vi "commandHandler.vi"(8 "error in (no error)":errorcluster, 10 "Camera":refnum<class>, 11 "CameraNetworkClient in":refnum<class "CameraNetworkServer.lvclass">) -> (0 "error out":errorcluster, 3 "CameraNetworkClient out":refnum<class "CameraNetworkServer.lvclass">)   [LabVIEW 2009, in "Hardware.lvlib" / "HWControllers.lvlib" / "CameraNetworkServer.lvclass"]
uses:
  CameraNetworkServer.lvclass
  Channels/Camera/Camera/Camera.lvclass
  CameraNetworkServer.lvclass/CameraNetworkServer.ctl
  Tools/CameraSettings/CamaraSettings.lvclass
  NetworkClient/NetworkServer.lvclass
panel:
  out "fps":dbl
  out "elements":T1(array[cluster])
  out "element":T2
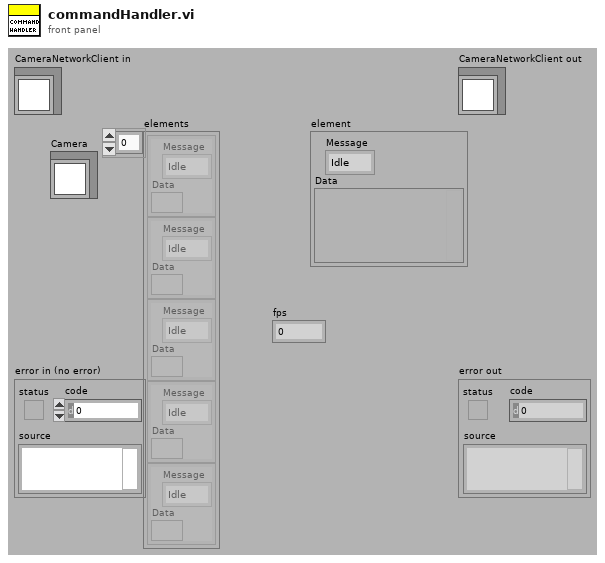
[diagram p1: front panel]
types:
  T1 = cluster{"Message":enum16{"Idle", "initialise", "configureAcquisition", "setTemperature", "getTemperature", "start", "stop", "sendImage", "close", "error", "ExitApp"}, "Data":variant}[]
  T2 = cluster{"Message":enum16{"Idle", "initialise", "configureAcquisition", "setTemperature", "getTemperature", "start", "stop", "sendImage", "close", "error", "ExitApp", "getAcquisitionStatus"}, "Data":variant}
  T3 = cluster{"CamaraSettings":refnum<class "CamaraSettings.lvclass">, "saveImages?":bool, "imagePaths":path[], "number of Images":i32}
  T4 = cluster{"Message":enum16{"Idle", "initialise", "configureAcquisition", "setTemperature", "getTemperature", "start", "stop", "sendImage", "close", "error", "ExitApp", "getAcquisitionStatus"}, bool}
  T5 = cluster{"cameraType":string, "imageName":string, "saved":string, "analysisType":string, "I16bit image data":i16[][], "path":path}
  T6 = cluster{"Message":enum16{"Idle", "initialise", "configureAcquisition", "setTemperature", "getTemperature", "start", "stop", "sendImage", "close", "error", "ExitApp", "getAcquisitionStatus"}, bool}[]
  T7 = cluster{"Message":enum16{"Idle", "initialise", "configureAcquisition", "setTemperature", "getTemperature", "start", "stop", "sendImage", "close", "error", "ExitApp"}, bool}
  T8 = enum16{"Idle", "initialise", "configureAcquisition", "setTemperature", "getTemperature", "start", "stop", "sendImage", "close", "error", "ExitApp"}
  T9 = cluster{"Message":enum16{"Idle", "initialise", "configureAcquisition", "setTemperature", "getTemperature", "start", "stop", "sendImage", "close", "error", "ExitApp", "getAcquisitionStatus"}, "Data":variant}[]
  T10 = enum16{"Idle", "initialise", "configureAcquisition", "setTemperature", "getTemperature", "start", "stop", "sendImage", "close", "error", "ExitApp", "getAcquisitionStatus"}
  T11 = cluster{"Message":enum16{"Idle", "initialise", "configureAcquisition", "setTemperature", "getTemperature", "start", "stop", "sendImage", "close", "error", "ExitApp"}, bool}[]
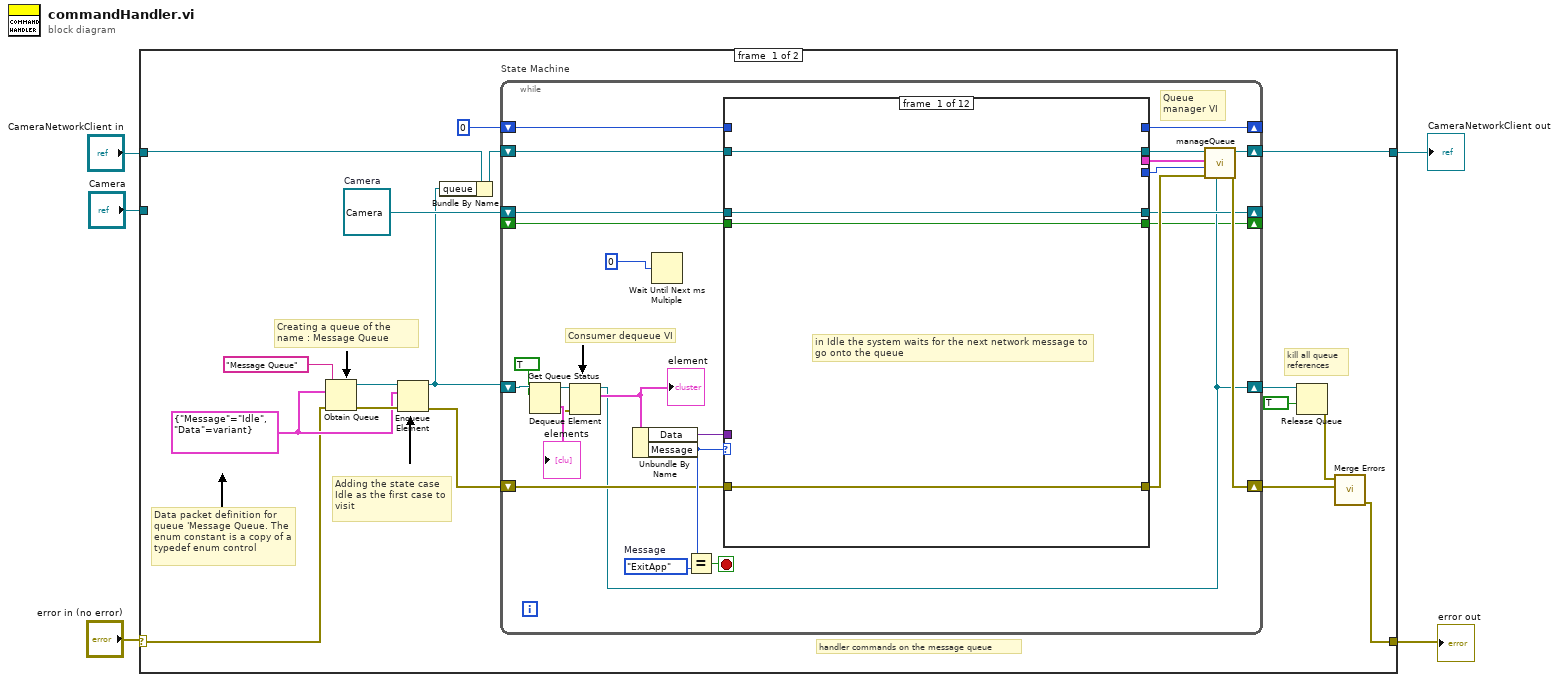
[diagram p0: block diagram]
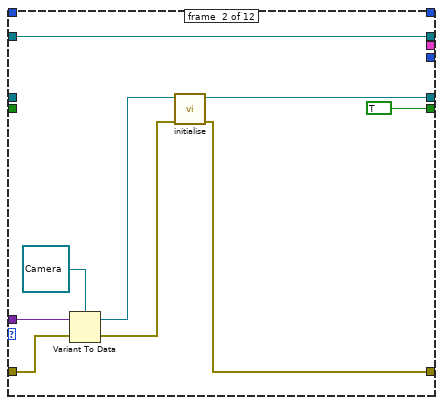
[diagram p2: hidden frame]
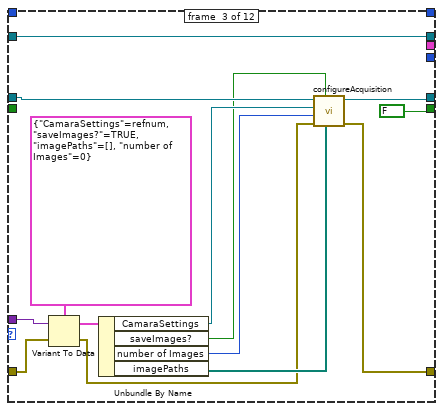
[diagram p3: hidden frame]
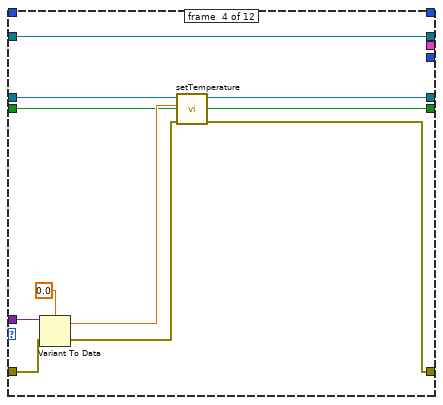
[diagram p4: hidden frame]
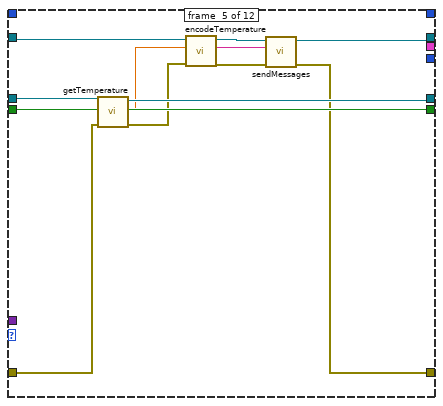
[diagram p5: hidden frame]
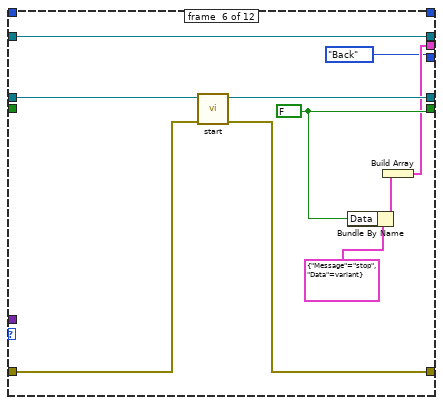
[diagram p6: hidden frame]
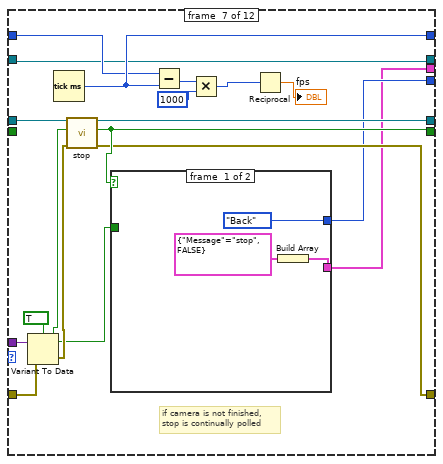
[diagram p7: hidden frame]
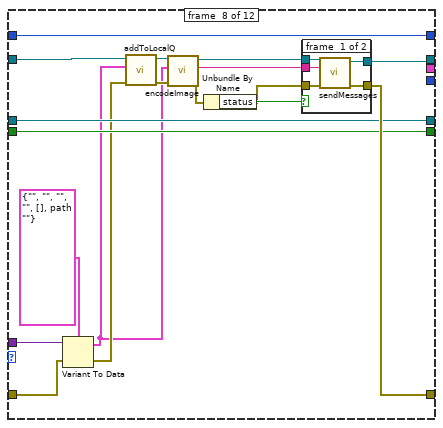
[diagram p9: hidden frame]
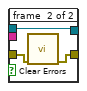
[diagram p10: hidden frame]
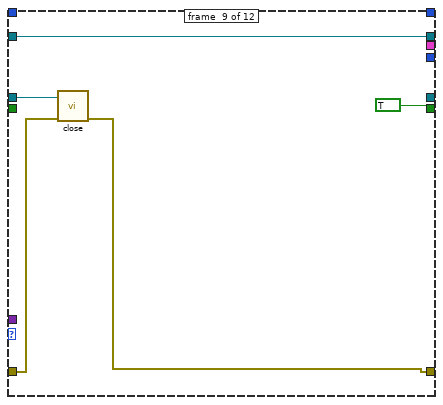
[diagram p11: hidden frame]
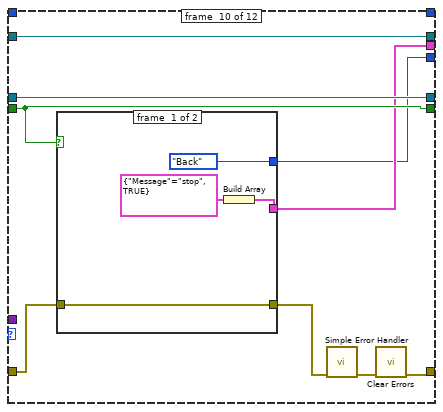
[diagram p12: hidden frame]
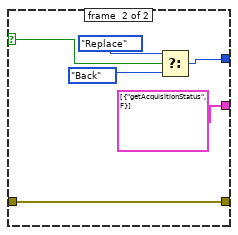
[diagram p13: hidden frame]
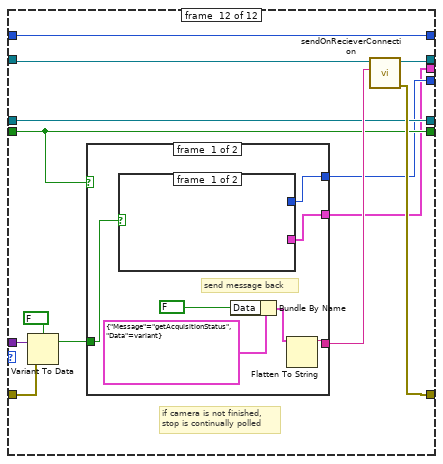
[diagram p15: hidden frame]
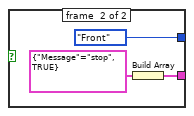
[diagram p16: hidden frame]
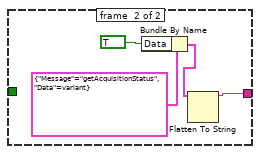
[diagram p17: hidden frame]
diagram:
  n1 = case shown="No Error" "error in (no error)" {
    selector: "error in (no error)" -> [w14 w210]
    tunnel: [w11 w210] -> w3
    tunnel: [w15 w209] -> w2
    tunnel: "CameraNetworkClient in" -> [w10 w209]
    tunnel: "Camera" -> [_ _]
    frame #0 {
      w8 = refnum<class "Camera.lvclass"> refnum  # Camera
      w17 = T2 {"Message"=enum."Idle", "Data"=variant}
      # "handler commands on the message queue"
      # "kill all queue \nreferences"
      # "Data packet definition for queue 'Message Queue. The enum constant is a copy of a typedef enum control"
      # "Adding the state case Idle as the first case to visit"
      # "Creating a queue of the name : Message Queue"
      n2 = Obtain Queue(name (unnamed)="Message Queue" ("Queue Name"), element data type=w17, error in (no error)=w14) -> (queue out=w20:refnum<queue>, error out=w21:errorcluster)  [unwired: 2 in, 1 out]
      n3 = Enqueue Element(queue=w20, element=w17, error in (no error)=w21) -> (queue out=w6:refnum<queue>, error out=w16:errorcluster)  [unwired: 1 in, 1 out]
      n4 = Bundle By Name(cluster=w10, "queue"=w6) -> (w9:refnum<class "CameraNetworkServer.lvclass">)
      n5 = while "State Machine" {
        shift-right: [w39] -> w12
        shift-left: w16 -> [w46]
        shift-right: [w34] -> w18
        shift-left: w6 -> [w30]
        shift-right: [w41] -> w15
        shift-left: w9 -> [w43]
        shift-right: [w36] -> _
        shift-left: w8 -> [w35]
        shift-right: [w33] -> _
        shift-left: _ -> [w32]
        shift-right: [w26] -> _
        shift-left: 0 -> [w25]
        stop <- w45 stop-if-true
        w37 = T8."ExitApp"  # Message
        # "Queue manager VI"
        # "Consumer dequeue VI"
        n6 = Get Queue Status(queue=w30, return elements? (F)=TRUE) -> (queue out=w31:refnum<queue>, error out=w27:errorcluster, elements=→"elements":T9)  [unwired: 1 in, 5 out]
        n7 = Dequeue Element(queue=w31, error in (no error)=w27) -> (queue out=w34:refnum<queue>, element=w44:T2)  [unwired: 1 in, 2 out]
        "element" <- w44
        n8 = Unbundle By Name(w44) -> ("Data"=w48:variant, "Message"=w47:T10)
        n9 = Wait Until Next ms Multiple(millisecond multiple=0) -> ()  [unwired: 1 out]
        n10 = Equal?(x=w47, y=w37) -> (x = y?=w45:bool)
        n11 = case shown="\"sendImage\"" w47 {
          tunnel: w46 -> [w50 w56 w73 w81 w95 w104 w120 w139 w156 w160 w178 w192]
          tunnel: [w50 w59 w63 w77 w86 w103 w110 w144 w157 w164 w178 w187] -> w40
          tunnel: w48 -> [_ w57 w74 w82 _ _ w122 w140 _ _ _ w194]
          tunnel: w43 -> [w52 w61 w75 w85 w93 w107 w111 w136 w154 w167 w181 w190]
          tunnel: [w52 w61 w75 w85 w91 w107 w111 w145 w154 w167 w181 w189] -> w42
          tunnel: [_ _ _ _ _ enum16{"Back", "Front", "Replace"}."Back" ("FNs") w109 _ _ w161 _ w183] -> w38
          tunnel: [_ _ _ _ _ w99 w108 _ _ w162 _ w182] -> w24
          tunnel: [w51 w60 w69 w83 w96 w105 w124 w141 _ w166 w179 w185] -> w36
          tunnel: w35 -> [w51 _ w70 w84 w97 w106 w125 w141 w158 w166 w179 w185]
          tunnel: [w49 TRUE ("stopped?") FALSE w76 w94 w101 w123 w138 TRUE w163 w180 w184] -> w33
          tunnel: w32 -> [w49 _ _ w76 w94 _ _ w138 _ w163 w180 w184]
          tunnel: [_ _ _ _ _ _ w117 w137 _ _ _ w186] -> w26
          tunnel: w25 -> [_ _ _ _ _ _ w116 w137 _ _ _ w186]
          frame #0 {
            # "in Idle the system waits for the next network message to \ngo onto the queue"
          }
          frame #1 {
            n12 = Variant To Data(error in=w56, Variant=w57, type=refnum<class "Camera.lvclass"> refnum ("Hardware:Channels.lvlib:Camera.lvclass")) -> (error out=w55:errorcluster, data=w53:refnum<class "Camera.lvclass">)
            n13 = call-dynamic "initialise.vi"("error in (no error)"=w55, "Camera in"=w53) -> ("error out"=w59:errorcluster, "Camera out"=w60:refnum<class "Camera.lvclass">)  [unwired: 8 in]
          }
          frame #2 {
            n14 = Variant To Data(error in=w73, Variant=w74, type=T3 {"CamaraSettings"=refnum, "saveImages?"=TRUE, "imagePaths"=[], "number of Images"=0}) -> (error out=w64:errorcluster, data=w71:T3)
            n15 = Unbundle By Name(w71) -> ("CamaraSettings"=w68:refnum<class "CamaraSettings.lvclass">, "saveImages?"=w67:bool, "number of Images"=w66:i32, "imagePaths"=w65:path[])
            n16 = call-dynamic "configureAcquisition.vi"("imagePaths"=w65, "saveImages?"=w67, "error in (no error)"=w64, "number of Images"=w66, "CameraSettings"=w68, "Camera in"=w70) -> ("error out"=w63:errorcluster, "Camera out"=w69:refnum<class "Camera.lvclass">)  [unwired: 4 in]
          }
          frame #3 {
            n17 = Variant To Data(error in=w81, Variant=w82, type=0.0 ("setPoint")) -> (error out=w80:errorcluster, data=w78:dbl)
            n18 = call-dynamic "setTemperature.vi"("error in (no error)"=w80, "setPoint"=w78, "Camera in"=w84) -> ("error out"=w77:errorcluster, "Camera out"=w83:refnum<class "Camera.lvclass">)  [unwired: 7 in]
          }
          frame #4 {
            n19 = call-dynamic "getTemperature.vi"("error in (no error)"=w95, "Camera in"=w97) -> ("error out"=w89:errorcluster, "temperature"=w88:dbl, "Camera out"=w96:refnum<class "Camera.lvclass">)  [unwired: 7 in]
            n20 = call "encodeTemperature.vi"("error in (no error)"=w89, "temperature"=w88, "CameraNetworkServer in"=w93) -> ("error out"=w90:errorcluster, "message"=w87:string, "CameraNetworkServer out"=w92:refnum<class "CameraNetworkServer.lvclass">)  [unwired: 6 in]
            n21 = call "sendMessages.vi"("error in (no error)"=w90, "messageString"=w87, "NetworkClient in"=w92) -> ("error out"=w86:errorcluster, "NetworkClient out"=w91:refnum<class "CameraNetworkServer.lvclass">)  [unwired: 7 in]
          }
          frame #5 {
            w101 = FALSE
            n22 = call-dynamic "start.vi"("error in (no error)"=w104, "Camera in"=w106) -> ("error out"=w103:errorcluster, "Camera out"=w105:refnum<class "Camera.lvclass">)  [unwired: 8 in]
            n23 = Bundle By Name(cluster=T2 {"Message"=enum."stop", "Data"=variant} ("element"), "Data"=w101) -> (w100:T2)
            n24 = Build Array(w100) -> (w99:T9)
          }
          frame #6 {
            # "if camera is not finished,\nstop is continually polled"
            n25 = Variant To Data(error in=w120, Variant=w122, type=TRUE) -> (error out=w119:errorcluster, data=w118:bool)
            n26 = Tick Count (ms)() -> (millisecond timer value=w117:u32)
            n27 = call-dynamic "stop.vi"("error in (no error)"=w119, "stop"=w118, "Camera in"=w125) -> ("error out"=w110:errorcluster, "stopped?"=w123:bool, "Camera out"=w124:refnum<class "Camera.lvclass">)  [unwired: 5 in, 1 out]
            n28 = case shown="False" w123 {
              tunnel: [w127 _] -> w108
              tunnel: [enum16{"Back", "Front", "Replace"}."Back" ("FNs") _] -> w109
              tunnel: w118 -> [_ _]
              frame #0 {
                n29 = Build Array(T4 {"Message"=enum."stop", FALSE}) -> (w127:T6)
              }
              frame #1 {
              }
            }
            n30 = Subtract(x=w116, y=w117) -> (x-y=w115:u32)
            n31 = Multiply(x=w115, y=1000) -> (x*y=w113:u32)
            n32 = Reciprocal(x=w113) -> (1/x=→"fps":dbl)
          }
          frame #7 {
            n33 = Variant To Data(error in=w139, Variant=w140, type=T5 {"cameraType"="", "imageName"="", "saved"="", "analysisType"="", "I16bit image data"=[], "path"=path ""} ("ImageData")) -> (error out=w133:errorcluster, data=w130:T5)
            n34 = call "addToLocalQ.vi"("error in (no error)"=w133, "ImageData"=w130, "CameraNetworkServer in"=w136) -> ("error out"=w134:errorcluster, "CameraNetworkServer out"=w135:refnum<class "CameraNetworkServer.lvclass">)  [unwired: 7 in]
            n35 = call "encodeImage.vi"("error in (no error)"=w134, "ImageData"=w130, "CameraNetworkClient in"=w135) -> ("error out"=w131:errorcluster, "MessageString"=w142:string, "CameraNetworkClient out"=w143:refnum<class "CameraNetworkServer.lvclass">)  [unwired: 6 in]
            n36 = Unbundle By Name(w131) -> ("status"=w132:bool)
            n37 = case shown="False" w132 {
              tunnel: [w150 w153] -> w145
              tunnel: [w149 w151] -> w144
              tunnel: w143 -> [w148 w153]
              tunnel: w142 -> [w147 _]
              tunnel: w131 -> [w146 w152]
              frame #0 {
                n38 = call "sendMessages.vi"("error in (no error)"=w146, "messageString"=w147, "NetworkClient in"=w148) -> ("error out"=w149:errorcluster, "NetworkClient out"=w150:refnum<class "CameraNetworkServer.lvclass">)  [unwired: 7 in]
              }
              frame #1 {
                n39 = call <vilib>:"Clear Errors.vi"("error in (no error)"=w152) -> ("error out"=w151:errorcluster)  [unwired: 6 in]
              }
            }
          }
          frame #8 {
            n40 = call-dynamic "close.vi"("error in (no error)"=w156, "Camera in"=w158) -> ("error out"=w157:errorcluster)  [unwired: 9 in]
          }
          frame #9 {
            n41 = case shown="True" w163 {
              selector: w163 -> [_ w172]
              tunnel: [w170 T6 [{"Message"=enum."getAcquisitionStatus", FALSE}]] -> w162
              tunnel: [enum16{"Back", "Front", "Replace"}."Back" ("FNs") w177] -> w161
              tunnel: w160 -> [w168 w173]
              tunnel: [w168 w173] -> w159
              frame #0 {
                n42 = Build Array(T4 {"Message"=enum."stop", TRUE}) -> (w170:T6)
              }
              frame #1 {
                n43 = Select(t=enum16{"Back", "Front", "Replace"}."Replace" ("FNs"), s=w172, f=enum16{"Back", "Front", "Replace"}."Back" ("FNs")) -> (s? t:f=w177:enum16{"Back", "Front", "Replace"})
              }
            }
            n44 = call <vilib>:"Simple Error Handler.vi"("error in (no error)"=w159) -> ("error out"=w165:errorcluster)  [unwired: 4 in, 4 out]
            n45 = call <vilib>:"Clear Errors.vi"("error in (no error)"=w165) -> ("error out"=w164:errorcluster)  [unwired: 6 in]
          }
          frame #10 {
          }
          frame #11 {
            # "if camera is not finished,\nstop is continually polled"
            n46 = Variant To Data(error in=w192, Variant=w194, type=FALSE) -> (data=w191:bool)  [unwired: 1 out]
            n47 = case shown="False" w184 {
              tunnel: [w201 _] -> w182
              tunnel: [w200 _] -> w183
              tunnel: w191 -> [w197 _]
              tunnel: [w199 w208] -> w188
              frame #0 {
                # "send message back"
                n48 = case shown="True" w197 {
                  tunnel: [_ w203] -> w201
                  tunnel: [_ enum16{"Back", "Front", "Replace"}."Front" ("FNs")] -> w200
                  frame #0 {
                  }
                  frame #1 {
                    n49 = Build Array(T7 {"Message"=enum."stop", TRUE}) -> (w203:T11)
                  }
                }
                n50 = Bundle By Name(cluster=T2 {"Message"=enum."getAcquisitionStatus", "Data"=variant}, "Data"=FALSE) -> (w195:T2)
                n51 = Flatten To String(anything=w195) -> (data string=w199:string)  [unwired: 3 in, 2 out]
              }
              frame #1 {
                n52 = Bundle By Name(cluster=T2 {"Message"=enum."getAcquisitionStatus", "Data"=variant}, "Data"=TRUE) -> (w205:T2)
                n53 = Flatten To String(anything=w205) -> (data string=w208:string)  [unwired: 3 in, 2 out]
              }
            }
            n54 = call "sendOnRecieverConnection.vi"("message"=w188, "NetworkServer in"=w190) -> ("error out"=w187:errorcluster, "NetworkServer out"=w189:refnum<class "CameraNetworkServer.lvclass">)  [unwired: 8 in]
          }
        }
        n55 = call "manageQueue.vi"("MessageQRef"=w34, "error in (no error)"=w40, "FNs"=w38, "Message"=w24, "CameraNetworkClient in"=w42) -> ("error out"=w39:errorcluster, "CameraNetworkClient out"=w41:refnum<class "CameraNetworkServer.lvclass">)  [unwired: 5 in]
      }
      n56 = Release Queue(queue=w18, force destroy? (F)=TRUE) -> (error out=w13:errorcluster)  [unwired: 1 in, 2 out]
      n57 = call <vilib>:"Merge Errors.vi"("error in 2 (no error)"=w12, "error in 1 (no error)"=w13) -> ("error out"=w11:errorcluster)  [unwired: 5 in]
    }
    frame #1 {
    }
  }
  "error out" <- w3
  "CameraNetworkClient out" <- w2
